vi "Get_Randomized_Image_Name-1.vi"(2 "error IN":errorcluster, 3 "Main Name":string) -> (0 "error OUT":errorcluster, 1 "Randomized name":string)   [LabVIEW 2017]
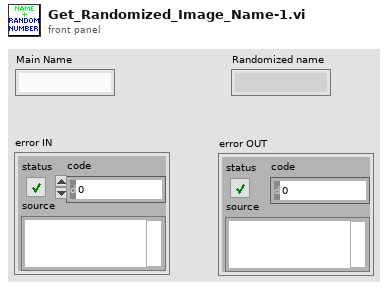
[diagram p1: front panel]
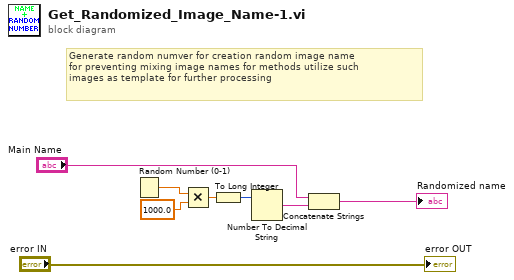
[diagram p0: block diagram]
diagram:
  # "Generate random numver for creation random image name \nfor preventing mixing image names for methods utilize such\nimages as template for further processing"
  n1 = Random Number (0-1)() -> (number: 0 to 1=w2:dbl)
  n2 = Multiply(x=w2, y=1000.0) -> (x*y=w1:dbl)
  n3 = To Long Integer(number=w1) -> (32bit integer=w5:i32)
  n4 = Number To Decimal String(number=w5) -> (decimal integer string=w4:string)  [unwired: 1 in]
  n5 = Concatenate Strings("Main Name", w4) -> (→"Randomized name":string)
  "error OUT" <- "error IN"
